vi "Sub_TimeString.vi"() -> ()   [LabVIEW 2018]
panel:
  out "日付/時間文字列":string
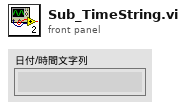
[diagram p1: front panel]
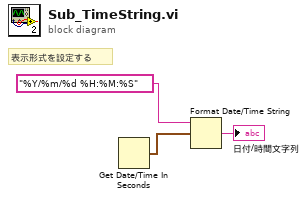
[diagram p0: block diagram]
diagram:
  # "表示形式を設定する"
  n1 = Get Date/Time In Seconds() -> (seconds since 1Jan1904=w3:timestamp)
  n2 = Format Date/Time String(time format string (%c)="%Y/%m/%d %H:%M:%S" ("時間形式文字列（%c）"), seconds (now)=w3) -> (date/time string=→"日付/時間文字列":string)  [unwired: 1 in]
